vi "Start DMM - Current Mode.vi"(8 "error in (no error)":errorcluster, 11 "Async Data out":T1={"Hardware"={"Switch Device"="", "DMM Device"="", "DMM -> Switch Trigger"=0, "Switch -> DMM Trigger"=0, "Sample Interval (sec)"=0.0, "Current Samples"=0, "Current Limit"=1.2, "Current Resolution"=5.5, "Auto-Read"=FALSE, "Keep Values"=FALSE}, "Communication"={"Status Q"=refnum, "Command Q"=refnum, "Voltage FIFO"=refnum, "Voltage Buffer"=[], "Current FIFO"=refnum, "Current Buffer"=[], "Async Events"=refnum}} {"Hardware"."Current Resolution" items=["3 1/2"=3.5, "4 1/2"=4.5, "5 1/2"=5.5, "6 1/2"=6.5, "7 1/2"=7.5]; "Hardware"."Sample Interval (sec)" format="%.2f"}) -> (0 "error out":errorcluster)   [LabVIEW 2011, in "Switch-DMM Custom Device.lvlib"]
uses:
  Switch-DMM Custom Device.lvlib
  Controls/Async Data.ctl
  Controls/Hardware.ctl
  <instrlib>/niDMM/nidmm.llb/niDMM Resolution in Digits.ctl
  Controls/Communication.ctl
  Controls/Async Status.ctl
  Controls/Async State.ctl
  Controls/Async Command.ctl
  Controls/Async Events.ctl
  <instrlib>/niDMM/nidmm.llb/niDMM Trigger.ctl
  <instrlib>/niDMM/nidmm.llb/niDMM Sample Trigger.ctl
  <instrlib>/niDMM/nidmm.llb/niDMM Function.ctl
  <instrlib>/niDMM/nidmm.llb/niDMM Configure Measurement Digits.vi
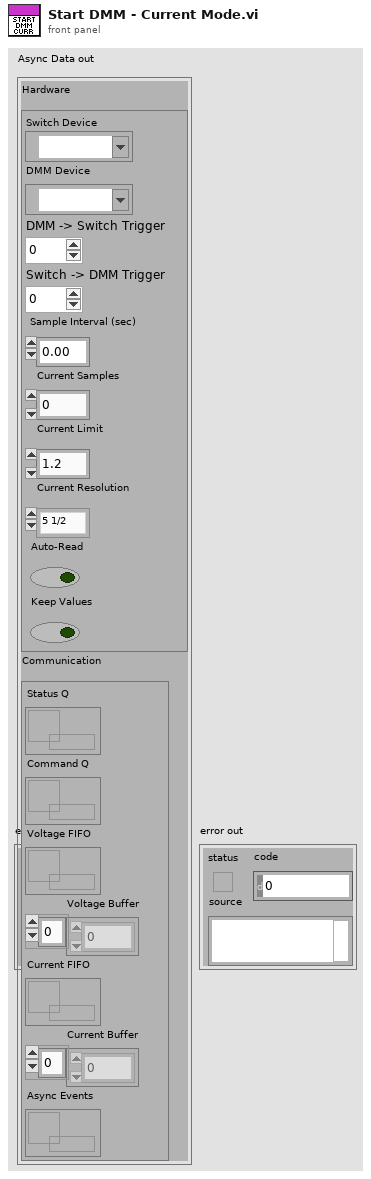
[diagram p1: front panel]
types:
  T1 = typedef "Switch-DMM Custom Device.lvlib/Async Data.ctl" = cluster{"Hardware":T2, "Communication":T4}
  T2 = typedef "Switch-DMM Custom Device.lvlib/Hardware.ctl" = cluster{"Switch Device":refnum<k15>, "DMM Device":refnum<k15>, "DMM -> Switch Trigger":u16, "Switch -> DMM Trigger":u16, "Sample Interval (sec)":dbl, "Current Samples":i32, "Current Limit":dbl, "Current Resolution":T3, "Auto-Read":bool, "Keep Values":bool}
  T3 = typedef "niDMM Resolution in Digits.ctl" = dbl
  T4 = typedef "Switch-DMM Custom Device.lvlib/Communication.ctl" = cluster{"Status Q":refnum<queue>, "Command Q":refnum<queue>, "Voltage FIFO":refnum<k33>, "Voltage Buffer":dbl[], "Current FIFO":refnum<k33>, "Current Buffer":dbl[], "Async Events":refnum<queue>}
  T5 = typedef "niDMM Trigger.ctl" = enum16{"Immediate", "External", "TTL 0", "TTL 1", "TTL 2", "TTL 3", "TTL 4", "TTL 5", "TTL 6", "Software", "TTL 7", "PXI Star", "LBR Trig 1", "Aux Trig 1"}
  T6 = typedef "niDMM Sample Trigger.ctl" = enum16{"Immediate", "External", "TTL 0", "TTL 1", "TTL 2", "TTL 3", "TTL 4", "TTL 5", "TTL 6", "Interval", "Software", "TTL 7", "PXI Star", "LBR Trig 1", "Aux Trig 1"}
  T7 = typedef "niDMM Function.ctl" = enum16{"DC Volts", "AC Volts", "DC Current", "AC Current", "2-wire Resistance", "4-wire Resistance", "Diode", "Frequency", "Period", "AC Volts DC Coupled", "Capacitance", "Inductance", "Temperature"}
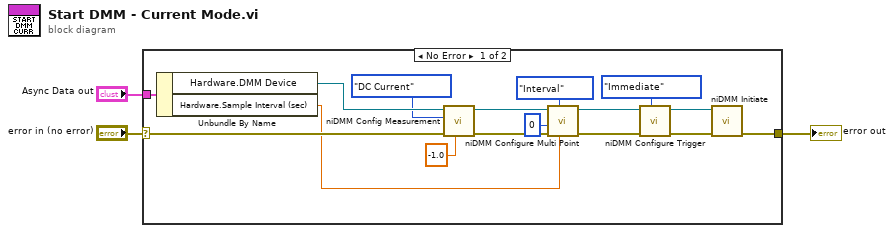
[diagram p0: block diagram]
diagram:
  n1 = case shown="No Error" "error in (no error)" {
    selector: "error in (no error)" -> [w5 w20]
    tunnel: [w19 w20] -> w3
    tunnel: "Async Data out" -> [w6 _]
    frame No Error {
      n2 = Unbundle By Name(w6) -> ("Hardware.DMM Device"=w18:refnum<k15>, "Hardware.Sample Interval (sec)"=w4:dbl)
      n3 = call-poly <instrlib>:"niDMM Config Measurement.vi"("Range"=-1.0, "error in (no error)"=w5, "Function"=niDMM_Function."DC Current", "instrument handle"=w18) -> ("error out"=w14:errorcluster, "instrument handle out"=w15:refnum<k15>)  [unwired: 6 in]
      n4 = call <instrlib>:"niDMM Configure Multi Point.vi"("Sample Interval (sec)"=w4, "Sample Trigger"=niDMM_Sample_Trigger."Interval", "error in (no error)"=w14, "Sample Count"=0, "instrument handle"=w15) -> ("error out"=w9:errorcluster, "instrument handle out"=w10:refnum<k15>)  [unwired: 5 in]
      n5 = call <instrlib>:"niDMM Configure Trigger.vi"("Trigger Source"=niDMM_Trigger."Immediate", "error in (no error)"=w9, "instrument handle"=w10) -> ("error out"=w7:errorcluster, "instrument handle out"=w8:refnum<k15>)  [unwired: 1 in, 6 out]
      n6 = call <instrlib>:"niDMM Initiate.vi"("error in (no error)"=w7, "instrument handle"=w8) -> ("error out"=w19:errorcluster)  [unwired: 8 in, 1 out]
    }
    frame Error {
    }
  }
  "error out" <- w3
